vi "NI6071E.ProcEvents.vi"(0 "i ref in":refnum<vi>, 5 "error in":errorcluster) -> (14 "i ref out":refnum<vi>, 19 "error out":errorcluster)   [LabVIEW 2014, in "NI6071E.lvlib"]
doc: "This method is used to define the events the object will listen to. Add your own events here."
uses:
  NI6071E.lvlib
  CSCore/BaseProcess/BaseProcess.event definition.ctl
  CSCore/CAEObj/CAEObj.event definition.ctl
  CSCore/BaseProcess/BaseProcess.descriptor string definition.ctl
  CSCore/BaseProcess/BaseProcess.lvlib
  CSCore/CAEObj/CAEObj.lvlib
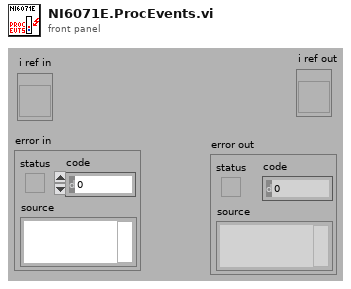
[diagram p1: front panel]
types:
  T1 = typedef "BaseProcess.lvlib/BaseProcess.event definition.ctl" = cluster{"CAEEvtDef":T2, "Data Descriptor":T3}
  T2 = typedef "CAEObj.lvlib/CAEObj.event definition.ctl" = cluster{"URL":string, "enable":bool, "ignoreResID":bool}
  T3 = typedef "BaseProcess.lvlib/BaseProcess.descriptor string definition.ctl" = string
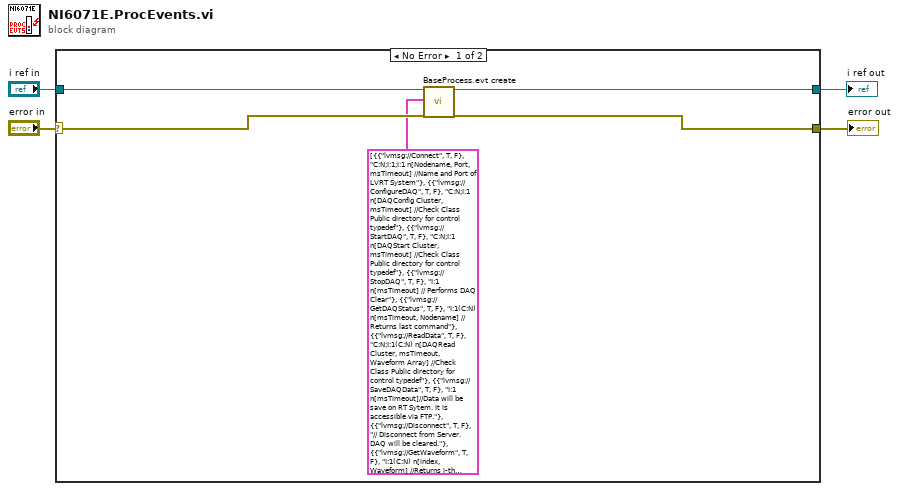
[diagram p0: block diagram]
diagram:
  n1 = case shown="No Error" "error in" {
    selector: "error in" -> [w6 w11]
    tunnel: "i ref in" -> [w9 w10]
    tunnel: [w8 w10] -> w3
    tunnel: [w7 w11] -> w2
    frame No Error {
      n2 = call "BaseProcess.evt create.vi"("i ref in"=w9, "newEvents"=T1[] [{"CAEEvtDef"={"URL"="lvmsg://Connect", "enable"=TRUE, "ignoreResID"=FALSE}, "Data Descriptor"="C:N;I:1;I:1 n[Nodename, Port, msTimeout] //Name and Port of LVRT System"}, {"CAEEvtDef"={"URL"="lvmsg://ConfigureDAQ", "enable"=TRUE, "ignoreResID"=FALSE}, "Data Descriptor"="C:N;I:1 n[DAQConfig Cluster, msTimeout] //Check Class Public directory for control typedef"}, {"CAEEvtDef"={"URL"="lvmsg://StartDAQ", "enable"=TRUE, "ignoreResID"=FALSE}, "Data Descriptor"="C:N;I:1 n[DAQStart Cluster, msTimeout] //Check Class Public directory for control typedef"}, {"CAEEvtDef"={"URL"="lvmsg://StopDAQ", "enable"=TRUE, "ignoreResID"=FALSE}, "Data Descriptor"="I:1 n[msTimeout] // Performs DAQ Clear"}, {"CAEEvtDef"={"URL"="lvmsg://GetDAQStatus", "enable"=TRUE, "ignoreResID"=FALSE}, "Data Descriptor"="I:1(C:N) n[msTimeout, Nodename] //Returns last command"}, {"CAEEvtDef"={"URL"="lvmsg://ReadData", "enable"=TRUE, "ignoreResID"=FALSE}, "Data Descriptor"="C:N;I:1(C:N) n[DAQRead Cluster, msTimeout, Waveform Array] //Check Class Public directory for control typedef"}, {"CAEEvtDef"={"URL"="lvmsg://SaveDAQData", "enable"=TRUE, "ignoreResID"=FALSE}, "Data Descriptor"="I:1 n[msTimeout]//Data will be save on RT Sytem. It is accessible via FTP."}, {"CAEEvtDef"={"URL"="lvmsg://Disconnect", "enable"=TRUE, "ignoreResID"=FALSE}, "Data Descriptor"="// Disconnect from Server. DAQ will be cleared."}, {"CAEEvtDef"={"URL"="lvmsg://GetWaveform", "enable"=TRUE, "ignoreResID"=FALSE}, "Data Descriptor"="I:1(C:N) n[index, Waveform] //Returns i-th waveform"}, {"CAEEvtDef"={"URL"="lvmsg://GetWaveforms", "enable"=TRUE, "ignoreResID"=FALSE}, "Data Descriptor"="(C:N) n[Waveforms] //Returns array of waveforms"}] ("new events(V3.0)"), "error in (no error)"=w6) -> ("i ref out"=w8:refnum<vi>, "error out"=w7:errorcluster)  [unwired: 13 in, 2 out]
    }
    frame Error {
    }
  }
  "i ref out" <- w3
  "error out" <- w2
